vi "Log_MessageHanlder_ListLogFiles.vi"(8 "error in (no error)":errorcluster, 11 "MessageHandler in":refnum<class "MessageHandler.lvclass">) -> (0 "error out":errorcluster, 1 "Log file paths":path[](array[path]), 2 "Log file nb":u32, 3 "MessageHandler out":refnum<class "MessageHandler.lvclass">)   [LabVIEW 2013, in "MessageHandler.lvclass"]
uses:
  MessageHandler.lvclass
  MessageHandler.lvclass/MessageHandler.ctl
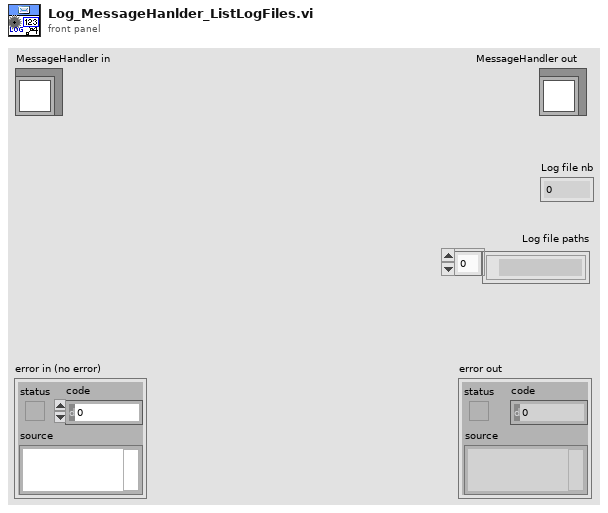
[diagram p1: front panel]
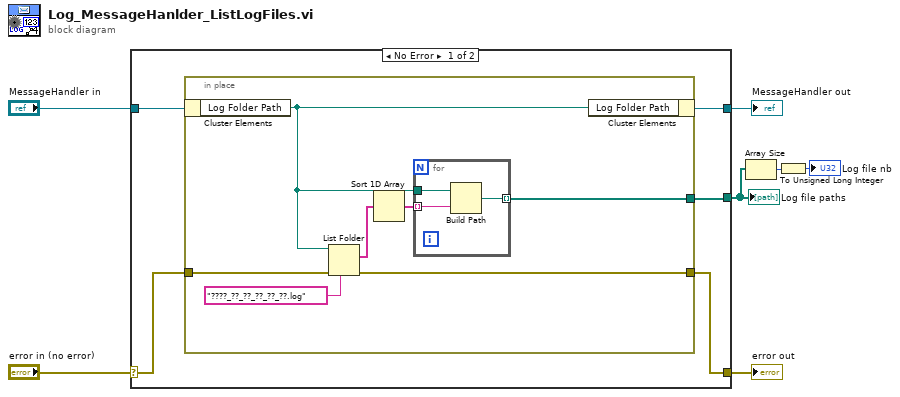
[diagram p0: block diagram]
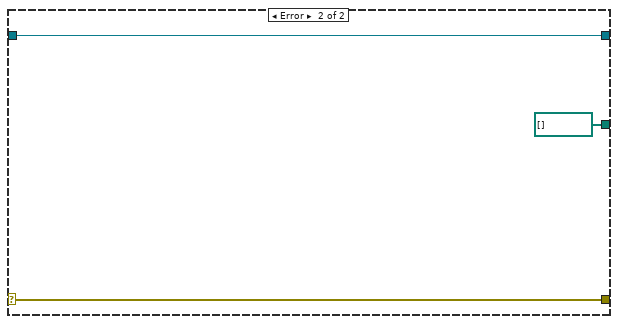
[diagram p2: hidden frame]
diagram:
  n1 = case shown="No Error" "error in (no error)" {
    selector: "error in (no error)" -> [w10 w25]
    tunnel: [w9 w25] -> w6
    tunnel: [w11 w24] -> w4
    tunnel: "MessageHandler in" -> [w12 w24]
    tunnel: [w8 path[] []] -> w3
    frame No Error {
      n2 = in-place {
        in-place-border: w10 -> [w15]
        in-place-border: [w14] -> w9
        in-place-border: [w13] -> w8
        n3 = in-place-cluster #1(w12) -> ("Log Folder Path"=w16:path)
        n4 = List Folder(path=w16, pattern="????_??_??_??_??_??.log", error in=w15) -> (filenames=w18:string[], error out=w14:errorcluster)  [unwired: 1 in, 2 out]
        n5 = Sort 1D Array(array=w18) -> (sorted array=w19:string[])
        n6 = for {
          tunnel: w19 -> [w21] mode=indexing
          tunnel: w16 -> [w22]
          tunnel: [w20] -> w13 mode=indexing
          n7 = Build Path(base path=w22, name or relative path=w21) -> (appended path=w20:path)
        }
        n8 = in-place-cluster #1("Log Folder Path"=w16) -> (w11:refnum<class "MessageHandler.lvclass">)
      }
    }
    frame Error {
    }
  }
  "error out" <- w6
  "MessageHandler out" <- w4
  "Log file paths" <- w3
  n9 = Array Size(array=w3) -> (size(s)=w2:i32)
  n10 = To Unsigned Long Integer(number=w2) -> (unsigned 32bit integer=→"Log file nb":u32)
